vi "Traverse_to_Traverse_Collision.vi"(5 "Current Position":sgl[](array[numeric])=[0.0, 100.0, 40.0] format="%.2f", 7 "Traverse Name":string, 8 "Model  Roll        Pitch       Yaw (deg)":sgl[](array[numeric]) format="%#.2f", 9 "Work in Tunnel Coordinates":T1, 10 "Simulate/Run":T2=enum."Run VI", 11 "New Position":sgl[](array[numeric])=[0.0, 100.0, 40.0] format="%.2f") -> (1 "Error String":string)   [LabVIEW 2014]
uses:
  Controls/User_Specific_mode.ctl
  Controls/Tunnel_Coordinates.ctl
  Route mapping/Exclude_cluster.ctl
  Route mapping/Box_size.ctl
  Route mapping/Exclusion_type.ctl
  Controls/Global_mode.ctl
  Route mapping/Pict_Plot_Axis.ctl
  Route mapping/Axis.ctl
  Globals/Preference_global.vi
  Globals/Trav_pos_global.vi
panel:
  out "Plan View":picture
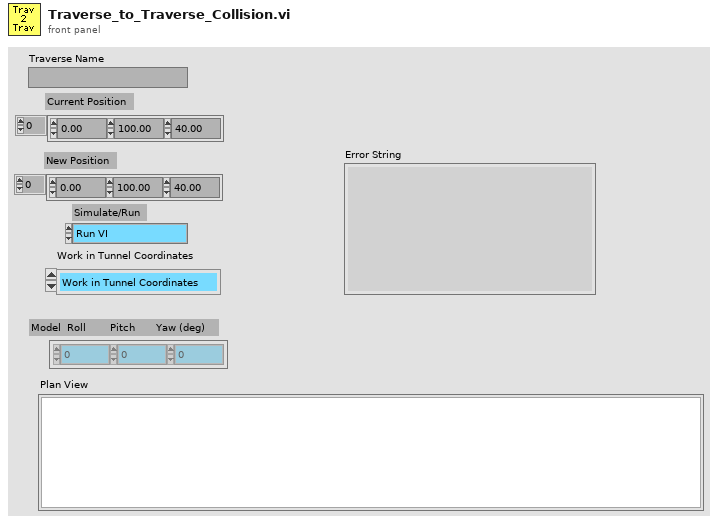
[diagram p1: front panel]
types:
  T1 = typedef "Tunnel_Coordinates.ctl" = enum16{"Work in Tunnel Coordinates", "Work in Model Coordinates"}
  T2 = typedef "User_Specific_mode.ctl" = enum16{"Check VI only", "Run VI"}
  T3 = typedef "Exclude_cluster.ctl" = cluster{"Sizes":T4, "Name":string, "Exclude Type":T5}
  T4 = typedef "Box_size.ctl" = cluster{"Max":sgl, "Min":sgl}[]
  T5 = typedef "Exclusion_type.ctl" = enum16{"Exclude completely", "Allow only vertical moves"}
  T6 = typedef "Global_mode.ctl" = enum16{"Read Global", "Load Global From File", "Write Global to File"}
  T7 = enum16{"Load setup from excel file", "Save setup to excel file"}
  T8 = typedef "Pict_Plot_Axis.ctl" = cluster{"Width":T9, "Height":T9}
  T9 = typedef "Axis.ctl" = enum16{"X Axis", "X Axis -ve", "Y Axis", "Y Axis -ve", "Z Axis", "Z Axis -ve"}
  T10 = typedef "Update_scan_value.ctl" = cluster{"Channel Name":string, "New Value":dbl}
  T11 = enum16{"To Traverse Coordinates", "To User Coordinates"}
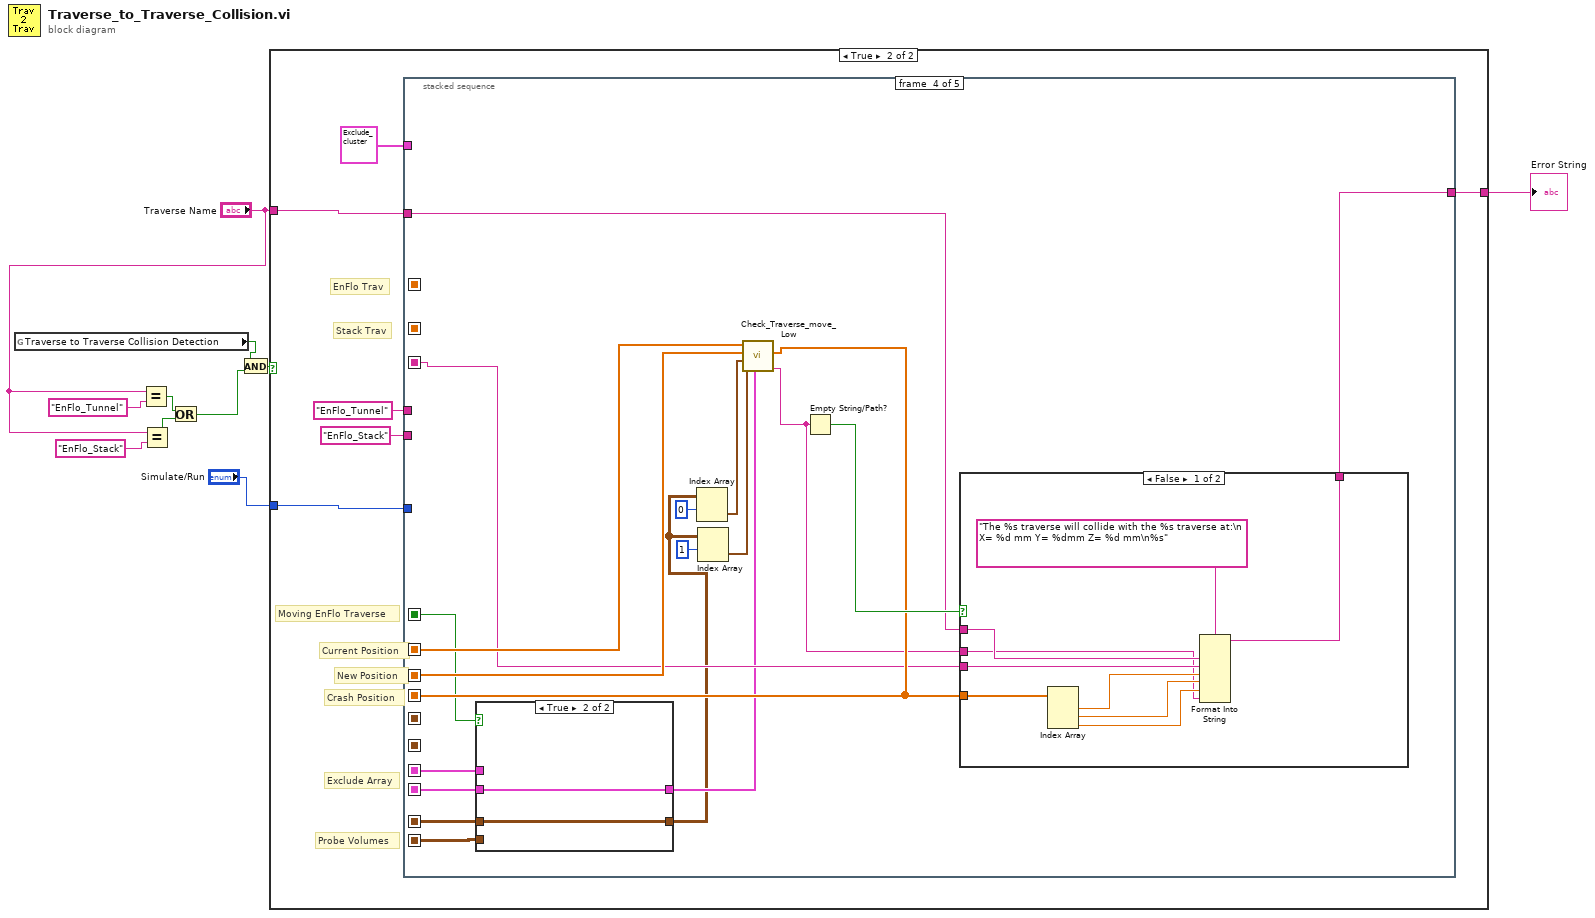
[diagram p0: block diagram]
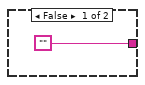
[diagram p2: hidden frame]
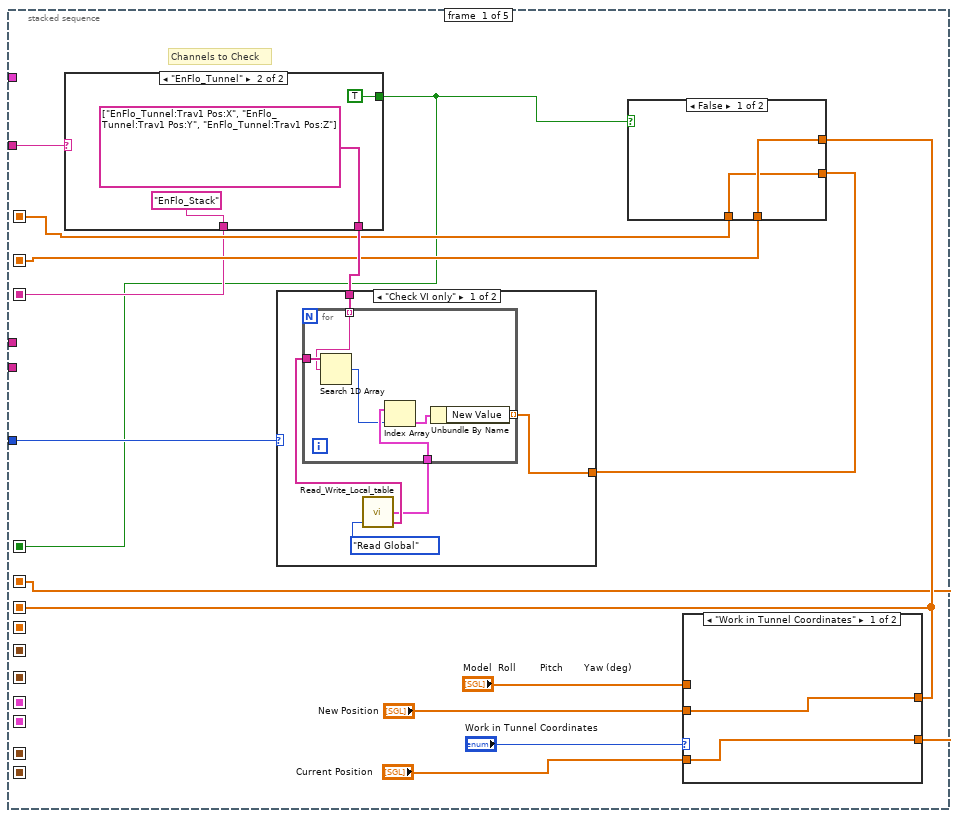
[diagram p3: hidden frame]
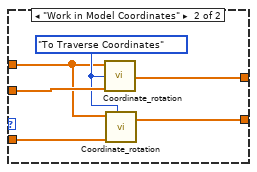
[diagram p5: hidden frame]
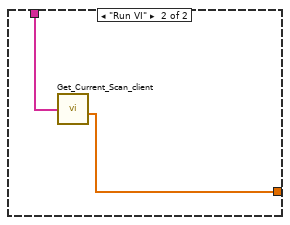
[diagram p6: hidden frame]
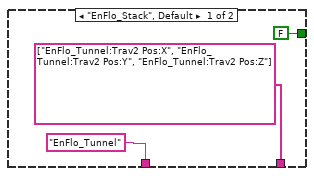
[diagram p7: hidden frame]
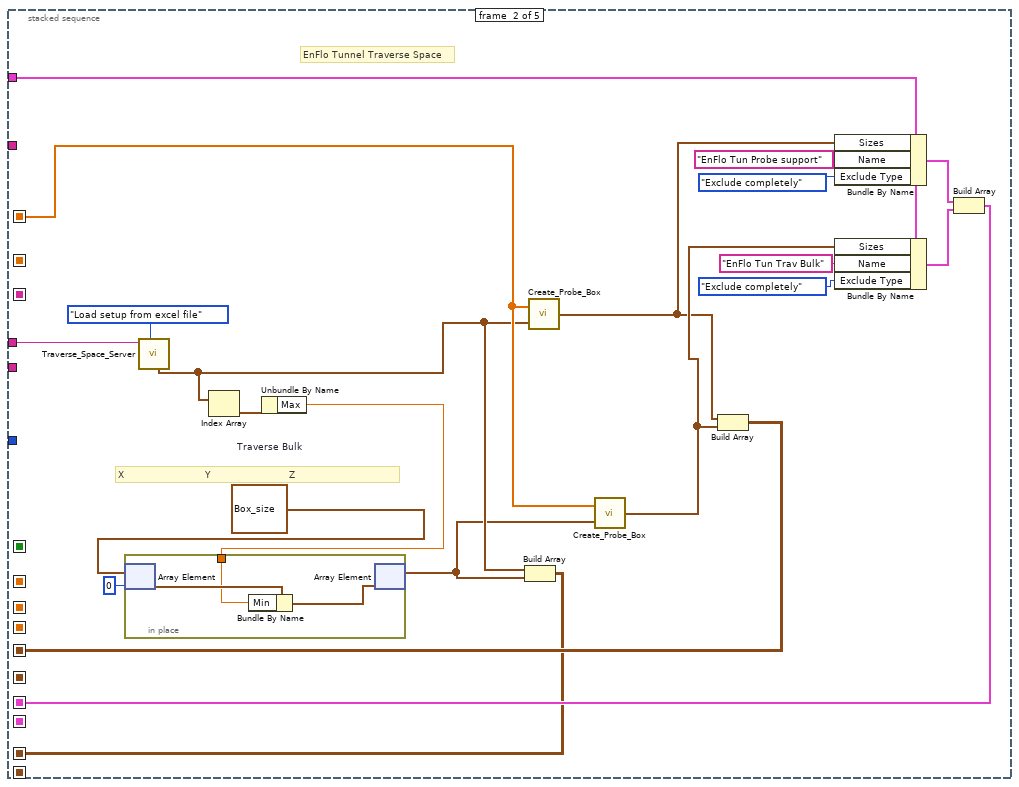
[diagram p8: hidden frame]
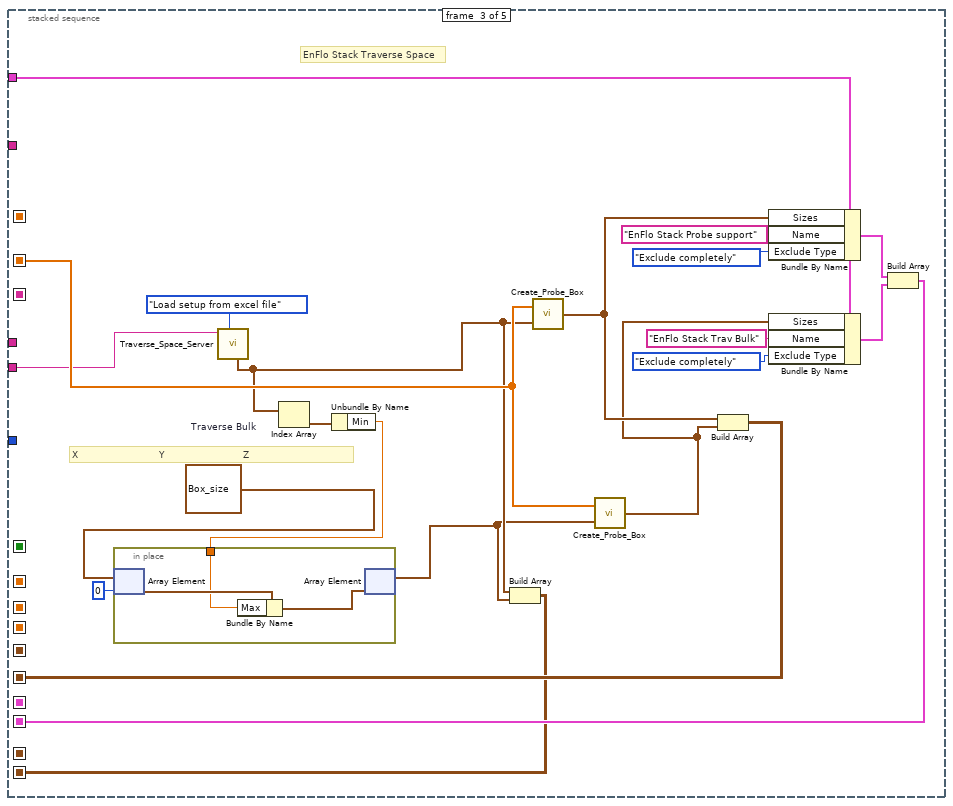
[diagram p9: hidden frame]
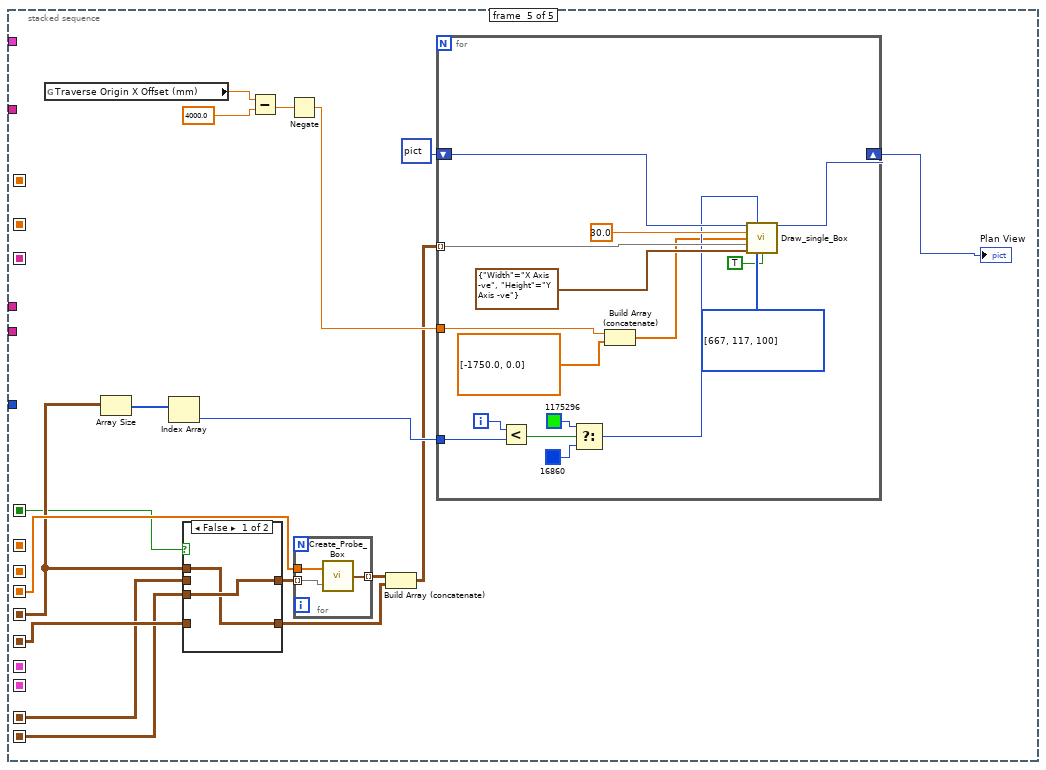
[diagram p12: hidden frame]
diagram:
  n1 = global read "Preference_global.vi" "Traverse to Traverse Collision Detection"() -> (w6:bool)
  n2 = Equal?(x="Traverse Name", y="EnFlo_Tunnel" ("Rig Setup")) -> (x = y?=w3:bool)
  n3 = Equal?(x="Traverse Name", y="EnFlo_Stack" ("Rig Setup")) -> (x = y?=w2:bool)
  n4 = Or(x=w3, y=w2) -> (x .or. y?=w1:bool)
  n5 = And(x=w6, y=w1) -> (x .and. y?=w7:bool)
  n6 = case shown="True" w7 {
    tunnel: "Traverse Name" -> [_ w17]
    tunnel: "Simulate/Run" -> [_ w16]
    tunnel: ["" w15] -> w8
    frame False {
    }
    frame True {
      # "Moving EnFlo Traverse"
      # "Exclude Array"
      # "Probe Volumes"
      # "Crash Position"
      # "Current Position"
      # "New Position"
      # "Stack Trav"
      # "EnFlo Trav"
      n7 = stacked-sequence {
        seq-local: [w25 _ _ _ _] -> [_ w83 _ _ _]
        seq-local: [w24 _ _ _ _] -> [_ _ w106 _ _]
        seq-local: [_ w82 _ _ _] -> [_ _ _ _ w145]
        seq-local: [_ _ w107 _ _] -> [_ _ _ _ w152]
        seq-local: [w22 _ _ _ _] -> [_ _ _ w124 _]
        seq-local: [w21 _ _ _ _] -> [_ _ _ w129 _]
        seq-local: [_ _ w97 _ _] -> [_ _ _ w121 _]
        seq-local: [_ w72 _ _ _] -> [_ _ _ w119 _]
        seq-local: [_ w71 _ _ _] -> [_ _ _ w120 w150]
        seq-local: [_ _ w95 _ _] -> [_ _ _ w118 w146]
        seq-local: [w19 _ _ _ _] -> [_ _ _ w128 _]
        seq-local: [_ _ _ w126 _] -> [_ _ _ _ w147]
        seq-local: [w18 _ _ _ _] -> [_ _ _ w116 w144]
        tunnel: w17 -> [w29 _ _ w125 _]
        tunnel: w16 -> [w31 _ _ _ _]
        tunnel: [_ _ _ w123 _] -> w15
        tunnel: T3 {"Sizes"=[{"Max"=15000.0, "Min"=0.0}, {"Max"=1000.0, "Min"=-1000.0}, {"Max"=300.0, "Min"=0.0}], "Name"="Roughness Elements", "Exclude Type"=enum."Allow only vertical moves"} ("Cluster") -> [_ w73 w96 _ _]
        tunnel: "EnFlo_Tunnel" -> [_ w70 _ _ _]
        tunnel: "EnFlo_Stack" -> [_ _ w93 _ _]
        frame #0 {
          # "Channels to Check"
          n8 = case shown="\"EnFlo_Tunnel\"" w29 {
            tunnel: [string[] ["EnFlo_Tunnel:Trav2 Pos:X", "EnFlo_Tunnel:Trav2 Pos:Y", "EnFlo_Tunnel:Trav2 Pos:Z"] string[] ["EnFlo_Tunnel:Trav1 Pos:X", "EnFlo_Tunnel:Trav1 Pos:Y", "EnFlo_Tunnel:Trav1 Pos:Z"]] -> w30
            tunnel: [FALSE TRUE] -> w18
            tunnel: ["EnFlo_Tunnel" "EnFlo_Stack"] -> w22
            frame "EnFlo_Stack", Default {
            }
            frame "EnFlo_Tunnel" {
            }
          }
          n9 = case shown="\"Check VI only\"" w31 {
            tunnel: [w44 w55] -> w23
            tunnel: w30 -> [w46 w56]
            frame "Check VI only" {
              n10 = call "Read_Write_Local_table.vi"("Mode"=Global_mode."Read Global") -> ("Ch Names"=w47:string[], "Ch Values Out"=w45:T10[])  [unwired: 2 in, 1 out]
              n11 = for {
                tunnel: w47 -> [w54]
                tunnel: w46 -> [w53] mode=indexing
                tunnel: w45 -> [w52]
                tunnel: [w49] -> w44 mode=indexing
                n12 = Search 1D Array(1D array=w54, element=w53) -> (index of element=w51:i32)  [unwired: 1 out]
                n13 = Index Array(array=w52, index=w51) -> (element=w50:T10)
                n14 = Unbundle By Name(w50) -> ("New Value"=w49:dbl)
              }
            }
            frame "Run VI" {
              n15 = call "Get_Current_Scan_client.vi"("ADAM Ch Names"=w56) -> ("Numerical Values"=w55:dbl[])  [unwired: 3 out]
            }
          }
          n16 = case shown="\"Work in Tunnel Coordinates\"" "Work in Tunnel Coordinates" {
            tunnel: "Model  Roll        Pitch       Yaw (deg)" -> [_ w40]
            tunnel: "New Position" -> [w37 w43]
            tunnel: [w37 w42] -> w21
            tunnel: "Current Position" -> [w36 w39]
            tunnel: [w36 w38] -> w19
            frame "Work in Tunnel Coordinates" {
            }
            frame "Work in Model Coordinates" {
              w41 = T11."To Traverse Coordinates" ("Mode")
              n17 = call "Coordinate_rotation.vi"("Model       Roll      Pitch       Yaw (deg)"=w40, "Input Position"=w43, "Mode"=w41) -> ("Output Position"=w42:sgl[])  [unwired: 2 in, 1 out]
              n18 = call "Coordinate_rotation.vi"("Model       Roll      Pitch       Yaw (deg)"=w40, "Input Position"=w39, "Mode"=w41) -> ("Output Position"=w38:sgl[])  [unwired: 2 in, 1 out]
            }
          }
          n19 = case shown="False" w18 {
            tunnel: [w32 w35] -> w25
            tunnel: w21 -> [w33 w35]
            tunnel: [w33 w34] -> w24
            tunnel: w23 -> [w32 w34]
            frame False {
            }
            frame True {
            }
          }
        }
        frame #1 {
          w66 = T4 [{"Max"=20000.0, "Min"=200.0}, {"Max"=3500.0, "Min"=-3500.0}, {"Max"=2000.0, "Min"=-2000.0}]  # Traverse Bulk
          # "X                           Y                          Z"
          # "EnFlo Tunnel Traverse Space"
          n20 = call "Traverse_Space_Server.vi"("Mode"=T7."Load setup from excel file", "Traverse Name"=w70) -> ("Probe Support Out"=w68:T4)  [unwired: 4 in, 5 out]
          n21 = Index Array(array=w68) -> (element=w67:cluster{"Max":sgl, "Min":sgl})  [unwired: 1 in]
          n22 = Unbundle By Name(w67) -> ("Max"=w63:sgl)
          n23 = in-place {
            in-place-border: w63 -> [w85]
            n24 = in-place-array #1(w66, 0) -> (w86:cluster{"Max":sgl, "Min":sgl})
            n25 = Bundle By Name(cluster=w86, "Min"=w85) -> (w84:cluster{"Max":sgl, "Min":sgl})
            n26 = in-place-array #1(w84) -> (w65:T4)  [unwired: 1 out]
          }
          n27 = Build Array(w68, w65) -> (w71:cluster{"Max":sgl, "Min":sgl}[][])
          n28 = call "Create_Probe_Box.vi"("Probe Volume"=w68, "Probe Position"=w83) -> ("Current Probe Volume"=w74:cluster{"Max":dbl, "Min":dbl}[])
          n29 = call "Create_Probe_Box.vi"("Probe Volume"=w65, "Probe Position"=w83) -> ("Current Probe Volume"=w75:cluster{"Max":dbl, "Min":dbl}[])
          n30 = Build Array(w74, w75) -> (w82:cluster{"Max":dbl, "Min":dbl}[][])
          n31 = Bundle By Name(cluster=w73, "Sizes"=w74, "Name"="EnFlo Tun Probe support", "Exclude Type"=Exclusion_type."Exclude completely") -> (w76:T3)
          n32 = Bundle By Name(cluster=w73, "Sizes"=w75, "Name"="EnFlo Tun Trav Bulk", "Exclude Type"=Exclusion_type."Exclude completely") -> (w77:T3)
          n33 = Build Array(w76, w77) -> (w72:T3[])
        }
        frame #2 {
          w90 = T4 [{"Max"=-200.0, "Min"=-20000.0}, {"Max"=3500.0, "Min"=-3500.0}, {"Max"=2000.0, "Min"=-2000.0}]  # Traverse Bulk
          # "X                           Y                          Z"
          # "EnFlo Stack Traverse Space"
          n34 = call "Traverse_Space_Server.vi"("Mode"=T7."Load setup from excel file", "Traverse Name"=w93) -> ("Probe Support Out"=w91:T4)  [unwired: 4 in, 5 out]
          n35 = Index Array(array=w91) -> (element=w92:cluster{"Max":sgl, "Min":sgl})  [unwired: 1 in]
          n36 = Unbundle By Name(w92) -> ("Min"=w88:sgl)
          n37 = in-place {
            in-place-border: w88 -> [w109]
            n38 = in-place-array #2(w90, 0) -> (w110:cluster{"Max":sgl, "Min":sgl})
            n39 = Bundle By Name(cluster=w110, "Max"=w109) -> (w108:cluster{"Max":sgl, "Min":sgl})
            n40 = in-place-array #2(w108) -> (w87:T4)  [unwired: 1 out]
          }
          n41 = Build Array(w91, w87) -> (w95:cluster{"Max":sgl, "Min":sgl}[][])
          n42 = call "Create_Probe_Box.vi"("Probe Volume"=w91, "Probe Position"=w106) -> ("Current Probe Volume"=w105:cluster{"Max":dbl, "Min":dbl}[])
          n43 = call "Create_Probe_Box.vi"("Probe Volume"=w87, "Probe Position"=w106) -> ("Current Probe Volume"=w101:cluster{"Max":dbl, "Min":dbl}[])
          n44 = Build Array(w105, w101) -> (w107:cluster{"Max":dbl, "Min":dbl}[][])
          n45 = Bundle By Name(cluster=w96, "Sizes"=w105, "Name"="EnFlo Stack Probe support", "Exclude Type"=Exclusion_type."Exclude completely") -> (w98:T3)
          n46 = Bundle By Name(cluster=w96, "Sizes"=w101, "Name"="EnFlo Stack Trav Bulk", "Exclude Type"=Exclusion_type."Exclude completely") -> (w99:T3)
          n47 = Build Array(w98, w99) -> (w97:T3[])
        }
        frame #3 {
          n48 = case shown="True" w116 {
            tunnel: [w131 w133] -> w122
            tunnel: w121 -> [_ w133]
            tunnel: [w130 w132] -> w111
            tunnel: w120 -> [_ w132]
            tunnel: w119 -> [w131 _]
            tunnel: w118 -> [w130 _]
            frame False {
            }
            frame True {
            }
          }
          n49 = Index Array(array=w111, index (row)=0) -> (element=w113:cluster{"Max":sgl, "Min":sgl}[])  [unwired: 1 in]
          n50 = Index Array(array=w111, index (row)=1) -> (element=w112:cluster{"Max":sgl, "Min":sgl}[])  [unwired: 1 in]
          n51 = call "Check_Traverse_move_Low.vi"("Exclude Array"=w122, "Probe Support"=w112, "Probe Volume"=w113, "New Position"=w129, "Current position"=w128) -> ("Error Comments"=w117:string, "Position At Crash"=w126:dbl[])  [unwired: 3 in]
          n52 = Empty String/Path?(string/path=w117) -> (empty?=w127:bool)
          n53 = case shown="False" w127 {
            tunnel: [w140 w143] -> w123
            tunnel: w117 -> [w134 w143]
            tunnel: w125 -> [w135 _]
            tunnel: w124 -> [w141 _]
            tunnel: w126 -> [w139 _]
            frame False {
              n54 = Index Array(array=w139) -> (element #1=w136:dbl, element #2=w138:dbl, element #3=w137:dbl)  [unwired: 3 in]
              n55 = Format Into String(format string="The %s traverse will collide with the %s traverse at:\n X= %d mm Y= %dmm Z= %d mm\n%s" ("Format String"), w135, w141, w136, w138, w137, w134) -> (resulting string=w140:string)  [unwired: 2 in, 1 out]
            }
            frame True {
            }
          }
        }
        frame #4 {
          n56 = global read "Trav_pos_global.vi" "Traverse Origin X Offset (mm)"() -> (w156:sgl)
          n57 = Array Size(array=w145) -> (size(s)=w159:i32[])
          n58 = Index Array(array=w159) -> (element=w158:i32)  [unwired: 1 in]
          n59 = case shown="False" w144 {
            tunnel: [w165 w168] -> w153
            tunnel: w152 -> [_ w168]
            tunnel: w150 -> [_ w167]
            tunnel: [w166 w167] -> w149
            tunnel: w146 -> [w166 _]
            tunnel: w145 -> [w165 _]
            frame False {
            }
            frame True {
            }
          }
          n60 = Subtract(x=w156, y=4000.0 ("x")) -> (x-y=w154:dbl)
          n61 = Negate(x=w154) -> (-x=w157:dbl)
          n62 = for {
            tunnel: w149 -> [w164] mode=indexing
            tunnel: [w163] -> w148 mode=indexing
            tunnel: w147 -> [w162]
            n63 = call "Create_Probe_Box.vi"("Probe Volume"=w164, "Probe Position"=w162) -> ("Current Probe Volume"=w163:cluster{"Max":dbl, "Min":dbl}[])
          }
          n64 = Build Array (concatenate)(w148, w153) -> (w151:cluster{"Max":dbl, "Min":dbl}[][])
          n65 = for {
            shift-right: [w181] -> w160
            shift-left: picture data[5B] ("Picture in") -> [w182]
            tunnel: w151 -> [w180] mode=indexing
            tunnel: w158 -> [w176]
            tunnel: w157 -> [w170]
            i -> [w177]
            n66 = Less?(x=w177, y=w176) -> (x < y?=w175:bool)
            n67 = Select(t=u32 1175296 ("color(black)"), s=w175, f=u32 16860 ("color(black)")) -> (s? t:f=w172:u32)
            n68 = Build Array (concatenate)(w170, dbl[] [-1750.0, 0.0] ("Min Values")) -> (w169:dbl[])
            n69 = call "Draw_single_Box.vi"("Picture in"=w182, "color(black)"=w172, "mm Per Pixel"=30.0, "Min Values"=w169, "Box Coordinates"=w180, "View"=T8 {"Width"=enum."X Axis -ve", "Height"=enum."Y Axis -ve"}, "Pixels per Axis"=i16[] [667, 117, 100], "fill?(F)"=TRUE) -> ("Picture out"=w181:picture)  [unwired: 7 out]
          }
          "Plan View" <- w160
        }
      }
    }
  }
  "Error String" <- w8
